vi "Convert Spectrum to Data Object and Display.vi"() -> ()   [LabVIEW 2017]
doc: "This VI converts the input spectrum into a data object that can be viewed on the Spectrum with Cursors XControl. Use the XControl to display magnitudes or phases of one or multiple channels of spectral data. This control displays the spectra on a graph and supports interactive data cursors. This XControl can be combined with other XControls to develop sophisticated user interfaces with minimal programming."
uses:
  <vilib>/addons/_XControls/Spectrum with Cursors/Spectrum with Cursors.xctl
  <vilib>/addons/_NISVFA/_Shared subVIs/Data Objects/Data/Data.lvclass
  <vilib>/addons/_NISVFA/_Shared subVIs/Data Objects/Data/Data.lvclass/Data.ctl
  <vilib>/addons/_NISVFA/_Shared subVIs/Data Objects/Y (DBL)/SV Convert Spectrum to Data Object.vi
  <vilib>/addons/_NISVFA/_Shared subVIs/Common/sv_Get NI Property Name String.vi
  <vilib>/addons/_NISVFA/_Shared subVIs/Data Objects/Data/Write Data Attributes.vi
  <vilib>/addons/_NISVFA/_Shared subVIs/Data Objects/Data/Read Data Attributes.vi
  <vilib>/addons/_NISVFA/_Shared subVIs/Data Objects/Y (DBL)/Y (1 Ch).lvclass
  C:/Program Files (x86)/National Instruments/LabVIEW 2017/vi.lib/addons/_NISVFA/_Shared subVIs/Data Objects/Data/Data.lvclass
  <vilib>/addons/_NISVFA/_Shared subVIs/Spectrum Info/sv_Convert Spectrum Info to Variant Attributes.vi
  <vilib>/addons/_NISVFA/_Shared subVIs/Data Objects/Y (DBL)/Write Y.vi
panel:
  out "Spectrum with Cursors":refnum<class "Data.lvclass">(xcontrol)
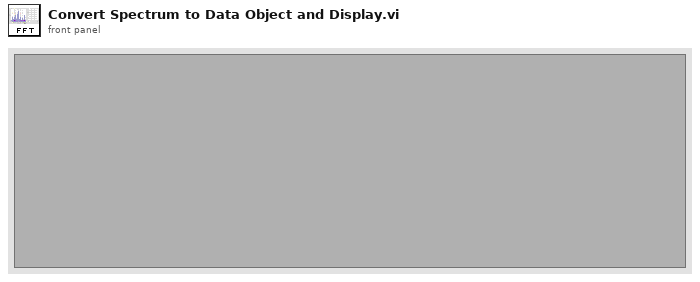
[diagram p1: front panel]
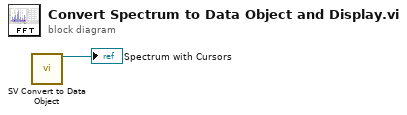
[diagram p0: block diagram]
diagram:
  n1 = call-poly <vilib>:"SV Convert to Data Object.vi"() -> ("Spectrum Data"=→"Spectrum with Cursors":refnum<class "Data.lvclass">)  [unwired: 18 in, 1 out]
